vi "EVEN校验.vi"(1 "校验字符串":string) -> (0 "校验码":string)   [LabVIEW 2014]
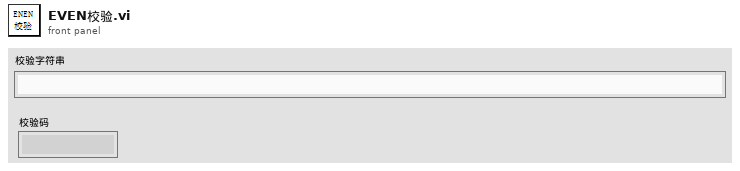
[diagram p1: front panel]
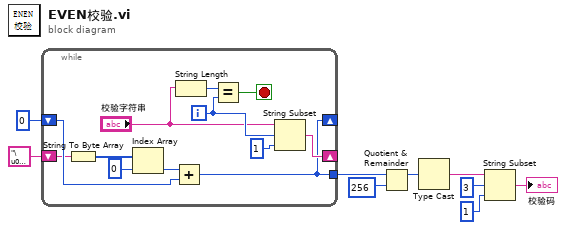
[diagram p0: block diagram]
diagram:
  n1 = while {
    shift-right: [w20] -> _
    shift-left: "\u0000" ("字符串") -> [w14]
    shift-right: [w15] -> _
    shift-left: 0 -> [w16]
    tunnel: [w15] -> w7
    i -> [w18]
    stop <- w17 stop-if-true
    n2 = String To Byte Array(string=w14) -> (unsigned byte array=w13:u8[])
    n3 = Index Array(array=w13, index=0 ("索引")) -> (element=w11:u8)
    n4 = Add(x=w11, y=w16) -> (x+y=w15:i32)
    n5 = String Length(string="校验字符串") -> (length=w19:i32)
    n6 = Equal?(x=w19, y=w18) -> (x = y?=w17:bool)
    n7 = String Subset(string="校验字符串", offset (0)=w18, length (rest)=1 ("长度（剩余）")) -> (substring=w20:string)
  }
  n8 = Quotient & Remainder(x=w7, y=256) -> (x-y*floor(x/y)=w5:i32)  [unwired: 1 out]
  n9 = Type Cast(x=w5) -> (*(type *) &x=w4:string)  [unwired: 1 in]
  n10 = String Subset(string=w4, offset (0)=3 ("偏移量(0)"), length (rest)=1 ("长度（剩余）")) -> (substring=→"校验码":string)
